vi "Begin.vi"(11 "Image Size":T1=enum."160x120") -> (0 "error out":errorcluster)   [LabVIEW 2012]
doc: "Called before other user functions, this VI is expected to open initial I/O refnums, load in file data, and do all program initialization. Notice that the <B>error out</B> terminal is simply used for data flow. Wiring it to other structures or subVIs ensures that this VI runs first."
uses:
  <vilib>/Rock Robotics/WPI/Camera/WPI_CameraImageSize.ctl
  <vilib>/Rock Robotics/WPI/DriverStation/WPI_DriverStationRobotMode2.ctl
  <vilib>/Rock Robotics/SystemInterfaces/DIO/FPGA_DIOPWMChannel.ctl
  <vilib>/Rock Robotics/SystemInterfaces/Typedef/FPGA_TypedefDigitalModule.ctl
  <vilib>/Rock Robotics/SystemInterfaces/DIO/FPGA_DIOChannel.ctl
  <vilib>/Rock Robotics/SystemInterfaces/DIO/FPGA_DIORelayChannel.ctl
  <vilib>/Rock Robotics/WPI/Joystick/WPI_JoystickDeviceEnum.ctl
  Robot Global Data.vi
  <vilib>/Rock Robotics/WPI/MotorControl/WPI_MotorControlOpen Talon.vi
  <vilib>/Rock Robotics/WPI/Compressor/WPI_CompressorGetSetRefNum.vi
  <vilib>/Rock Robotics/WPI/Camera/WPI_CameraWhite Balance Values.ctl
  <vilib>/Rock Robotics/WPI/Camera/WPI_CameraExposure Values.ctl
  <vilib>/Rock Robotics/WPI/Camera/WPI_CameraFrameRate.ctl
  <vilib>/Rock Robotics/SystemInterfaces/Typedef/FPGA_TypedefSolenoidModule.ctl
  <vilib>/Rock Robotics/WPI/Solenoid/WPI_SolenoidChannel.ctl
  <vilib>/Rock Robotics/WPI/Counter/WPI_CounterDigitalInputToDigitalSource.vi
  <vilib>/Rock Robotics/WPI/Encoder/WPI_EncoderType.ctl
  <vilib>/Rock Robotics/WPI/Solenoid/WPI_SolenoidOpenSingle.vi
panel:
  out "error out 3":errorcluster
  out "error out 2":errorcluster
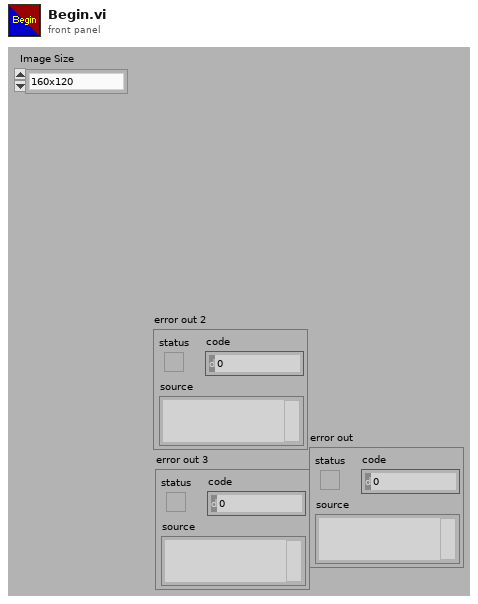
[diagram p1: front panel]
types:
  T1 = typedef "WPI_CameraImageSize.ctl" = enum16{"640x480", "320x240", "160x120"}
  T2 = typedef "WPI_DriverStationRobotMode2.ctl" = enum16{"Autonomous Disabled", "Autonomous Enabled", "Teleop Disabled", "Teleop Enabled", "Timeout", "Finish", "Test Disabled", "Test Enabled"}
  T3 = typedef "FPGA_DIOPWMChannel.ctl" = enum8{"PWM 1", "PWM 2", "PWM 3", "PWM 4", "PWM 5", "PWM 6", "PWM 7", "PWM 8", "PWM 9", "PWM 10", "Invalid"}
  T4 = typedef "FPGA_TypedefDigitalModule.ctl" = enum16{"Digital Module 1", "Digital Module 2"}
  T5 = typedef "FPGA_DIORelayChannel.ctl" = enum8{"Relay 1", "Relay 2", "Relay 3", "Relay 4", "Relay 5", "Relay 6", "Relay 7", "Relay 8", "Invalid"}
  T6 = typedef "FPGA_DIOChannel.ctl" = enum8{"DIO 1", "DIO 2", "DIO 3", "DIO 4", "DIO 5", "DIO 6", "DIO 7", "DIO 8", "DIO 9", "DIO 10", "DIO 11", "DIO 12", "DIO 13", "DIO 14", "Invalid"}
  T7 = typedef "WPI_SolenoidChannel.ctl" = enum8{"Solenoid 1", "Solenoid 2", "Solenoid 3", "Solenoid 4", "Solenoid 5", "Solenoid 6", "Solenoid 7", "Solenoid 8", "Invalid"}
  T8 = typedef "FPGA_TypedefSolenoidModule.ctl" = enum16{"Solenoid Module 1", "Solenoid Module 2"}
  T9 = typedef "WPI_EncoderType.ctl" = enum16{"1x", "2x", "4x"}
  T10 = typedef "WPI_JoystickDeviceEnum.ctl" = enum16{"USB 1", "USB 2", "USB 3", "USB 4", "Kinect 1", "Kinect 2"}
  T11 = typedef "WPI_CameraFrameRate.ctl" = u32
  T12 = typedef "WPI_CameraExposure Values.ctl" = enum16{"Auto", "Flicker-free 50 Hz", "Flicker-free 60 Hz", "Hold current"}
  T13 = typedef "WPI_CameraWhite Balance Values.ctl" = enum16{"Auto", "Fixed indoor", "Fixed outdoor 1", "Fixed outdoor 2", "Fixed fluorescent 1", "Fixed fluorescent 2", "Hold current"}
  T14 = typedef "WPI_MotorControlDeviceRef.ctl" = cluster{"DeviceStatus":errorcluster, "Type":enum16{"PWM", "CAN"}, "PWM":cluster{"Digital Module":T4, "PWM Channel":T3, "DeadBand":T15}, "CAN":cluster{"Device Number":u8, "Control Mode":T16, "Semaphore":T17, "Max Vout":dbl}, "Invert":bool, "TransformRef":T18, "InvTransformRef":T18}
  T15 = typedef "WPI_PWMDeadband.ctl" = cluster{"Name":string, "maxPositivePwm":i32, "minPositivePwm":i32, "centerPwm":i32, "maxNegativePwm":i32, "minNegativePwm":i32, "angularRange":u16}
  T16 = typedef "WPI_CANJaguar_ControlMode.ctl" = enum8{"Percent VBus", "Current", "Speed", "Position", "Voltage"}
  T17 = typedef "Semaphore RefNum" = refnum<k1>
  T18 = typedef "WPI_PWMTransform_ConPane.ctl" = refnum<vi>
  T19 = typedef "WPI_CompressorDevRef.ctl" = cluster{"DevStatus":errorcluster, "DigitalInputDevRef":T20, "RelayDevRef":T21}
  T20 = typedef "WPI_DigitalInputDevRef.ctl" = cluster{"DevStatus":errorcluster, "DIO Channel":T6, "Digital Module":T4}
  T21 = typedef "WPI_RelayDevRef.ctl" = cluster{"DevStatus":errorcluster, "Relay Channel":T5, "Digital Module":T4, "Relay Direction":T22}
  T22 = typedef "WPI_RelayDirection.ctl" = enum16{"Both directions", "Forward only", "Reverse only"}
  T23 = typedef "WPI_SolenoidDevRef.ctl" = cluster{"DevStatus":errorcluster, "Solenoid Module":T8, "Forward Solenoid Channel":T7, "Reverse Solenoid Channel":T7}
  T24 = typedef "FPGA_CounterEncoderSourceConvertionLVSourceType.ctl" = cluster{"DevStatus":errorcluster, "AnalogTriggerMode?":bool, "DigitalMode":cluster{"Digital Module":T4, "DIO Channel":T25}, "AnalogTriggerMode":cluster{"AnalogTriggerIndex":T26, "OutputType":T27}}
  T25 = typedef "FPGA_DIODigitalSourceChannel.ctl" = enum8{"DIO 1", "DIO 2", "DIO 3", "DIO 4", "DIO 5", "DIO 6", "DIO 7", "DIO 8", "DIO 9", "DIO 10", "DIO 11", "DIO 12", "DIO 13", "DIO 14", "Disabled"}
  T26 = typedef "FPGA_AnalogTriggerIndex.ctl" = enum8{"Trig 0", "Trig 1", "Trig 2", "Trig 3", "Trig 4", "Trig 5", "Trig 6", "Trig 7", "Invalid"}
  T27 = typedef "FPGA_AnalogTriggerOutType.ctl" = enum16{"InWindow", "TriggerState", "Rising", "Falling"}
  T28 = typedef "WPI_EncoderDevRef.ctl" = cluster{"DevStatus":errorcluster, "EncoderIndex":T29, "CounterIndex":T30, "DistancePerCount":dbl, "Decoding Type":T9}
  T29 = typedef "FPGA_EncoderIdx.ctl" = enum8{"Enc 0", "Enc 1", "Enc 2", "Enc 3", "Invalid"}
  T30 = typedef "FPGA_CounterCtrSystemIndex.ctl" = enum8{"Ctr 0", "Ctr 1", "Ctr 2", "Ctr 3", "Ctr 4", "Ctr 5", "Ctr 6", "Ctr 7", "Invalid"}
  T31 = typedef "WPI_JoystickDevRef.ctl" = cluster{"Device":T10}
  T32 = typedef "WPI_CameraDevRef.ctl" = cluster{"Camera Address":string, "CameraStatus":errorcluster, "Acquire Image Notifier":refnum<notifier>}
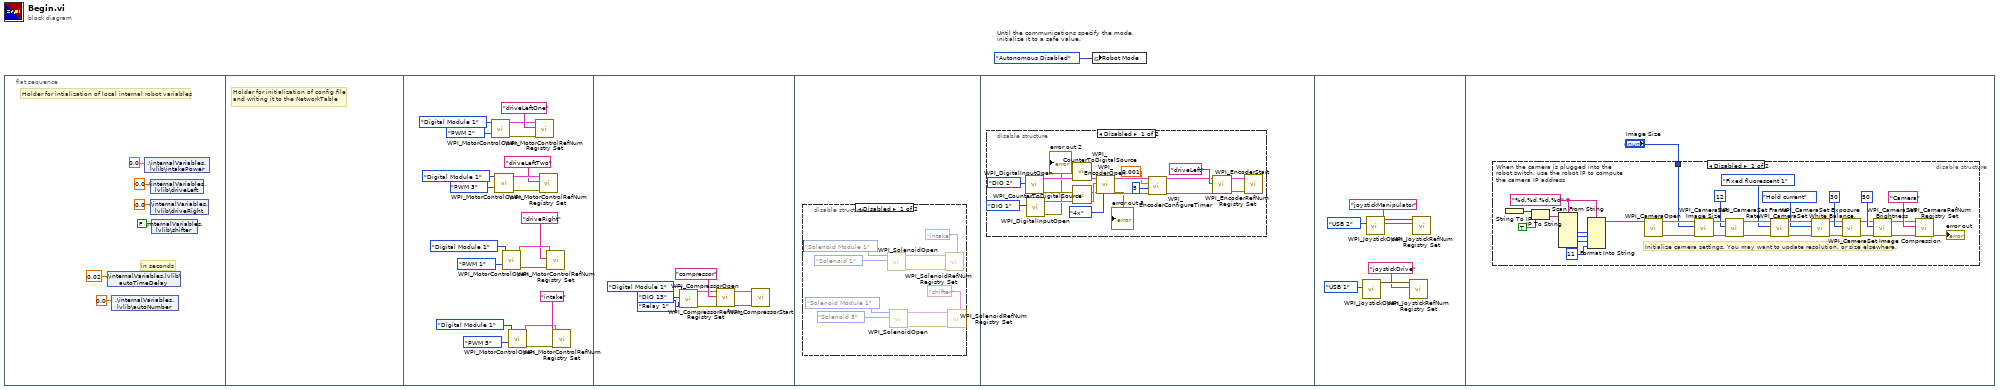
[diagram p0: block diagram]
diagram:
  # "Until the communications specify the mode,\ninitialize it to a safe value."
  n1 = flat-sequence {
    frame #0 {
      # "in seconds"
      # "Holder for intialization of local internal robot variables"
      n2 = shared-variable ".\\internalVariables.lvlib\\autoTimeDelay"(0.02 ("autoTimeDelay")) -> ()  [unwired: 1 in, 1 out]
      n3 = shared-variable ".\\internalVariables.lvlib\\autoNumber"(0.0 ("autoTimeDelay")) -> ()  [unwired: 1 in, 1 out]
      n4 = shared-variable ".\\internalVariables.lvlib\\intakePower"(0.0 ("driveLeft")) -> ()  [unwired: 1 in, 1 out]
      n5 = shared-variable ".\\internalVariables.lvlib\\driveLeft"(0.0 ("driveLeft")) -> ()  [unwired: 1 in, 1 out]
      n6 = shared-variable ".\\internalVariables.lvlib\\driveRight"(0.0 ("driveRight")) -> ()  [unwired: 1 in, 1 out]
      n7 = shared-variable ".\\internalVariables.lvlib\\shifter"(FALSE ("shifter")) -> ()  [unwired: 1 in, 1 out]
    }
    frame #1 {
      # "Holder for initialization of config file\nand writing it to the NetworkTable"
    }
    frame #2 {
      n8 = call-poly <vilib>:"WPI_MotorControlOpen.vi"("PWM Channel"=FPGA_DIOPWMChannel."PWM 2", "Digital Module (Module 1)"=FPGA_TypedefDigitalModule."Digital Module 1") -> ("error out"=w14:errorcluster, "MotorControlDeviceRef"=w13:T14)  [unwired: 8 in]
      n9 = call-poly <vilib>:"WPI_MotorControlOpen.vi"("PWM Channel"=FPGA_DIOPWMChannel."PWM 3", "Digital Module (Module 1)"=FPGA_TypedefDigitalModule."Digital Module 1") -> ("error out"=w21:errorcluster, "MotorControlDeviceRef"=w22:T14)  [unwired: 8 in]
      n10 = call-poly <vilib>:"WPI_MotorControlOpen.vi"("PWM Channel"=FPGA_DIOPWMChannel."PWM 1", "Digital Module (Module 1)"=FPGA_TypedefDigitalModule."Digital Module 1") -> ("error out"=w26:errorcluster, "MotorControlDeviceRef"=w27:T14)  [unwired: 8 in]
      n11 = call-poly <vilib>:"WPI_MotorControlOpen.vi"("PWM Channel"=FPGA_DIOPWMChannel."PWM 5", "Digital Module (Module 1)"=FPGA_TypedefDigitalModule."Digital Module 1") -> ("error out"=w9:errorcluster, "MotorControlDeviceRef"=w8:T14)  [unwired: 8 in]
      n12 = call <vilib>:"WPI_MotorControlRefNum Registry Set.vi"("error in (no error)"=w14, "refnum name"="driveLeftOne", "MotorControlDevRef"=w13) -> ()  [unwired: 7 in, 2 out]
      n13 = call <vilib>:"WPI_MotorControlRefNum Registry Set.vi"("error in (no error)"=w21, "refnum name"="driveLeftTwo", "MotorControlDevRef"=w22) -> ()  [unwired: 7 in, 2 out]
      n14 = call <vilib>:"WPI_MotorControlRefNum Registry Set.vi"("error in (no error)"=w26, "refnum name"="driveRight", "MotorControlDevRef"=w27) -> ()  [unwired: 7 in, 2 out]
      n15 = call <vilib>:"WPI_MotorControlRefNum Registry Set.vi"("error in (no error)"=w9, "refnum name"="intake", "MotorControlDevRef"=w8) -> ()  [unwired: 7 in, 2 out]
    }
    frame #3 {
      n16 = call <vilib>:"WPI_CompressorOpen.vi"("Pressure Switch DIO Channel"=FPGA_DIOChannel."DIO 13", "Relay Digital Module (Module 1)"=FPGA_TypedefDigitalModule."Digital Module 1", "Relay Channel"=FPGA_DIORelayChannel."Relay 1") -> ("CompressorDevRef"=w30:T19, "error out"=w28:errorcluster)  [unwired: 11 in]
      n17 = call <vilib>:"WPI_CompressorRefNum Registry Set.vi"("error in (no error)"=w28, "refnum name"="compressor", "CompressorDevRef"=w30) -> ("error out"=w32:errorcluster, "CompressorDevRef"=w31:T19)  [unwired: 7 in]
      n18 = call <vilib>:"WPI_CompressorStart.vi"("error in (no error)"=w32, "CompressorDevRef"=w31) -> ()  [unwired: 8 in, 2 out]
    }
    frame #4 {
      n19 = disable-structure shown="Disabled" {
        frame Disabled {
          n20 = call-poly <vilib>:"WPI_SolenoidOpen.vi"("Solenoid Channel"=WPI_SolenoidChannel."Solenoid 1" ("Forward Solenoid Channel"), "Solenoid Module (Module 1)"=FPGA_TypedefSolenoidModule."Solenoid Module 1") -> ("error out"=w40:errorcluster, "SolenoidDevRef"=w39:T23)  [unwired: 8 in]
          n21 = call-poly <vilib>:"WPI_SolenoidOpen.vi"("Solenoid Channel"=WPI_SolenoidChannel."Solenoid 3" ("Forward Solenoid Channel"), "Solenoid Module (Module 1)"=FPGA_TypedefSolenoidModule."Solenoid Module 1") -> ("error out"=w41:errorcluster, "SolenoidDevRef"=w42:T23)  [unwired: 8 in]
          n22 = call <vilib>:"WPI_SolenoidRefNum Registry Set.vi"("error in (no error)"=w40, "refnum name"="intake", "SolenoidDevRef"=w39) -> ()  [unwired: 7 in, 2 out]
          n23 = call <vilib>:"WPI_SolenoidRefNum Registry Set.vi"("error in (no error)"=w41, "refnum name"="shifter", "SolenoidDevRef"=w42) -> ()  [unwired: 7 in, 2 out]
        }
        frame Enabled {
        }
      }
    }
    frame #5 {
      n24 = disable-structure shown="Disabled" {
        frame Disabled {
          n25 = call <vilib>:"WPI_DigitalInputOpen.vi"("DIO Channel"=FPGA_DIOChannel."DIO 2") -> ("error out"=w48:errorcluster, "DigitalInputDevRef"=w61:T20)  [unwired: 9 in]
          "error out 3" <- w48
          n26 = call <vilib>:"WPI_DigitalInputOpen.vi"("DIO Channel"=FPGA_DIOChannel."DIO 1") -> ("error out"=→"error out 2":errorcluster, "DigitalInputDevRef"=w62:T20)  [unwired: 9 in]
          n27 = call-poly <vilib>:"WPI_CounterToDigitalSource.vi"("DigitalInputDevRef"=w61) -> ("Digital Source"=w58:T24)  [unwired: 6 in]
          n28 = call-poly <vilib>:"WPI_CounterToDigitalSource.vi"("DigitalInputDevRef"=w62) -> ("Digital Source"=w57:T24)  [unwired: 6 in]
          n29 = call <vilib>:"WPI_EncoderOpen.vi"("Decoding Type"=WPI_EncoderType."4x", "error in (no error)"=w48, "BSource"=w57, "ASource"=w58) -> ("error out"=w54:errorcluster, "EncoderDevRef"=w55:T28)  [unwired: 6 in]
          n30 = call <vilib>:"WPI_EncoderConfigureTimer.vi"("error in (no error)"=w54, "Number Samples to Average"=u8 5, "Minimum Rate"=0.001, "EncoderDevRef"=w55) -> ("error out"=w51:errorcluster, "EncoderDevRef"=w52:T28)  [unwired: 6 in]
          n31 = call <vilib>:"WPI_EncoderRefNum Registry Set.vi"("error in (no error)"=w51, "refnum name"="driveLeft", "EncoderDevRef"=w52) -> ("error out"=w49:errorcluster, "EncoderDevRef"=w50:T28)  [unwired: 7 in]
          n32 = call <vilib>:"WPI_EncoderStart.vi"("error in (no error)"=w49, "EncoderDevRef"=w50) -> ()  [unwired: 8 in, 2 out]
        }
        frame Enabled {
        }
      }
    }
    frame #6 {
      n33 = call <vilib>:"WPI_JoystickOpen.vi"("JoystickDevice"=WPI_JoystickDeviceEnum."USB 1") -> ("JoystickDevRef"=w68:T31)  [unwired: 10 in]
      n34 = call <vilib>:"WPI_JoystickOpen.vi"("JoystickDevice"=WPI_JoystickDeviceEnum."USB 2") -> ("JoystickDevRef"=w65:T31)  [unwired: 10 in]
      n35 = call <vilib>:"WPI_JoystickRefNum Registry Set.vi"("refnum name"="joystickDrive", "JoystickDevRef"=w68) -> ()  [unwired: 8 in, 2 out]
      n36 = call <vilib>:"WPI_JoystickRefNum Registry Set.vi"("refnum name"="joystickManipulator", "JoystickDevRef"=w65) -> ()  [unwired: 8 in, 2 out]
    }
    frame #7 {
      n37 = disable-structure shown="Disabled" {
        disable-tunnel: "Image Size" -> [w71 _]
        frame Disabled {
          w74 = "%d.%d.%d.%d" ("format string")
          # "When the camera is plugged into the\nrobot switch, use the robot IP to compute\nthe camera IP address"
          # "Initialize camera settings. You may want to update resolution, or size elsewhere."
          n38 = String To IP() -> (0:w81:u32)  [unwired: 1 in]
          n39 = IP To String(1:TRUE ("dot notation? (F)"), 2:w81) -> (0:w79:string)
          n40 = Scan From String(format string=w74, input string=w79) -> (output 1=w78:i32, output 2=w77:i32, output 3=w76:i32)  [unwired: 7 in, 3 out]
          n41 = Format Into String(format string=w74, w78, w77, w76, 11 ("Compression")) -> (resulting string=w73:string)  [unwired: 2 in, 1 out]
          n42 = call <vilib>:"WPI_CameraOpen.vi"("Camera Address"=w73) -> ("error out"=w92:errorcluster, "CameraDevRef"=w93:T32)  [unwired: 1 in, 8 out]
          n43 = call <vilib>:"WPI_CameraSet Image Size.vi"("error in (no error)"=w92, "Image Size"=w71, "CameraDevRef"=w93) -> ("error out"=w91:errorcluster, "CameraDevRef Out"=w94:T32)  [unwired: 7 out]
          n44 = call <vilib>:"WPI_CameraSet Frame Rate.vi"("error in (no error)"=w91, "Frame Rate (fps)"=T11 12, "CameraDevRef"=w94) -> ("error out"=w90:errorcluster, "CameraDevRef Out"=w96:T32)  [unwired: 7 out]
          n45 = call <vilib>:"WPI_CameraSet White Balance.vi"("error in (no error)"=w90, "White Balance"=WPI_CameraWhite_Balance_Values."Fixed fluorescent 1", "CameraDevRef"=w96) -> ("error out"=w89:errorcluster, "CameraDevRef Out"=w95:T32)  [unwired: 7 out]
          n46 = call <vilib>:"WPI_CameraSet Exposure.vi"("error in (no error)"=w89, "Exposure"=WPI_CameraExposure_Values."Hold current", "CameraDevRef"=w95) -> ("error out"=w88:errorcluster, "CameraDevRef Out"=w98:T32)  [unwired: 7 out]
          n47 = call <vilib>:"WPI_CameraSet Image Compression.vi"("error in (no error)"=w88, "Compression"=30, "CameraDevRef"=w98) -> ("error out"=w87:errorcluster, "CameraDevRef Out"=w97:T32)  [unwired: 7 out]
          n48 = call <vilib>:"WPI_CameraSet Brightness.vi"("error in (no error)"=w87, "Brightness"=50, "CameraDevRef"=w97) -> ("error out"=w85:errorcluster, "CameraDevRef Out"=w86:T32)  [unwired: 7 out]
          n49 = call <vilib>:"WPI_CameraRefNum Registry Set.vi"("error in (no error)"=w85, "refnum name"="Camera", "CameraDevRef"=w86) -> ("error out"=→"error out":errorcluster)  [unwired: 8 out]
        }
        frame Enabled {
        }
      }
    }
  }
  n50 = global write "Robot Global Data.vi" "Robot Mode"(WPI_DriverStationRobotMode2."Autonomous Disabled" ("Robot Mode")) -> ()
